vi "Pre Launch Init.vi"(11 "Test Executive Builder View in":refnum<class "Test Executive Builder View.lvclass">) -> (0 "error out":errorcluster, 3 "Test Executive Builder View out":refnum<class "Test Executive Builder View.lvclass">)   [LabVIEW 2017, in "Test Executive Builder View.lvclass"]
doc: "(<B>Filename</B>: Actor Framework.lvlib:Actor.lvclass:Pre Launch Init.vi)\n\nDefines behavior that occurs after the Launch Nested Actor method is invoked but before the actor's Actor Core method begins running.\n\nBy default, this method does nothing. A descendant class may override it to define behavior."
uses:
  Test Executive Builder View.lvclass
  <vilib>/gpm_packages/@cs/mva-viewable/Source/IViewable/IViewable/IViewable.lvclass
  <vilib>/ActorFramework/Actor/Actor.lvclass
  Test Executive Builder View Messages/Register Msg/Test Executive Builder View Register Msg.lvclass
  C:/Program Files (x86)/National Instruments/LabVIEW 2017/vi.lib/ActorFramework/Actor/Actor.lvclass
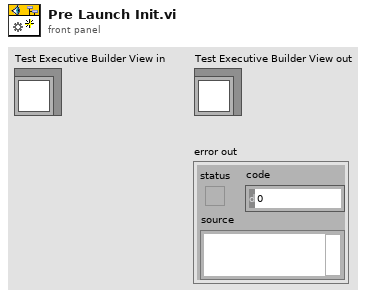
[diagram p1: front panel]
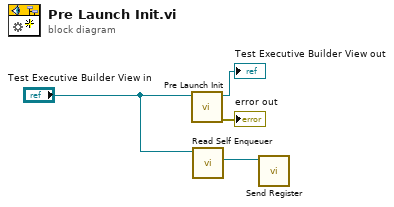
[diagram p0: block diagram]
diagram:
  n1 = call-parent "Pre Launch Init.vi"("IViewable in"="Test Executive Builder View in") -> ("error out"=→"error out":errorcluster, "IViewable out"=→"Test Executive Builder View out":refnum<class "Test Executive Builder View.lvclass">)  [unwired: 9 in]
  n2 = call <vilib>:"Read Self Enqueuer.vi"("Actor"="Test Executive Builder View in") -> ("Self Enqueuer"=w1:refnum<class "Message Enqueuer.lvclass">)  [unwired: 10 in]
  n3 = call "Send Register.vi"("Message Enqueuer"=w1) -> ()  [unwired: 9 in, 2 out]
